vi "Upg4,5_datainsamling.vi"() -> ()   [LabVIEW 2024]
panel:
  out "Mätvärden":dbl[](array[numeric])
  in  "stanna pump":bool
  in  "Samplingsintervall (ms)":dbl
  in  "avsluta mätning":bool
  in  "Konstant (m/V)":dbl
  # "Skriv in konstant bestämd i upg 3"
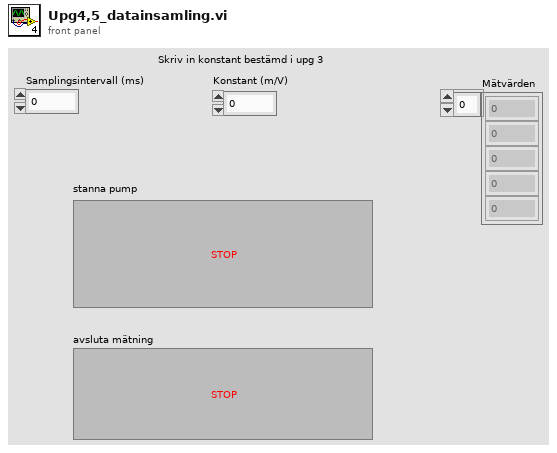
[diagram p1: front panel]
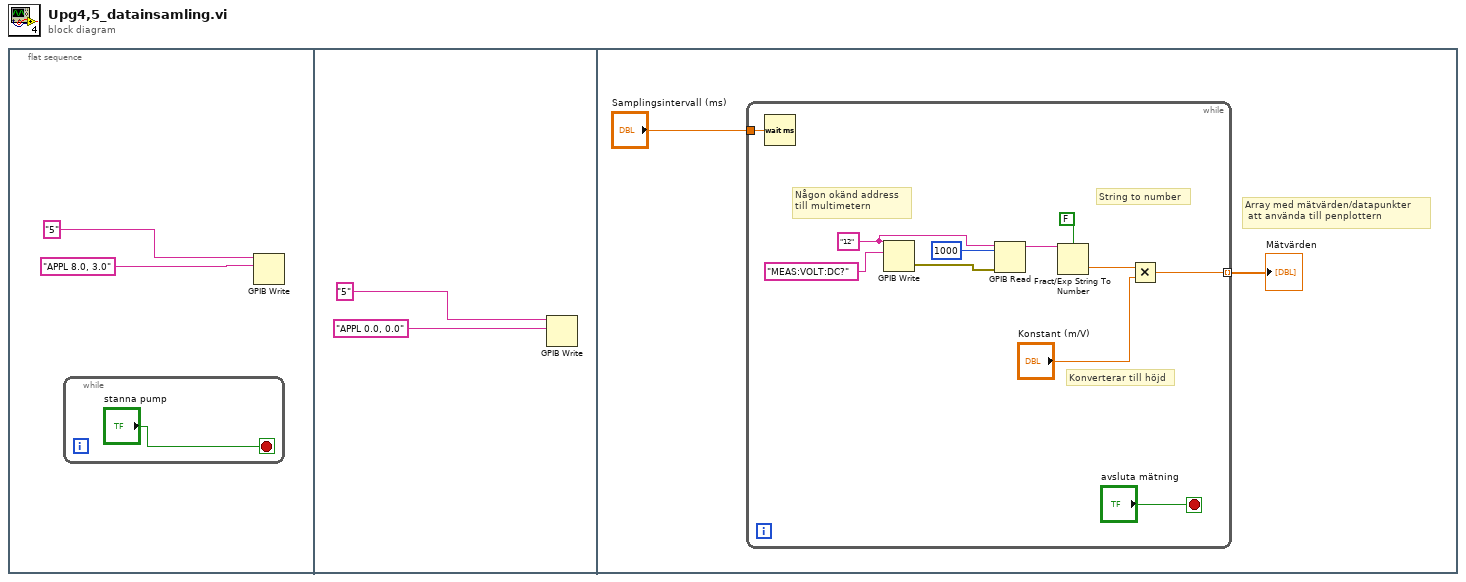
[diagram p0: block diagram]
diagram:
  n1 = flat-sequence {
    frame #0 {
      n2 = while {
        stop <- "stanna pump" stop-if-true
      }
      n3 = GPIB Write(0:"5" ("address string"), 1:"APPL 8.0, 3.0" ("data")) -> ()  [unwired: 3 in, 2 out]
    }
    frame #1 {
      n4 = GPIB Write(0:"5" ("address string"), 1:"APPL 0.0, 0.0" ("data")) -> ()  [unwired: 3 in, 2 out]
    }
    frame #2 {
      # "Array med mätvärden/datapunkter\n att använda till penplottern"
      n5 = while {
        tunnel: [w11] -> w6 mode=indexing
        tunnel: "Samplingsintervall (ms)" -> [w9]
        stop <- "avsluta mätning" stop-if-true
        w16 = "12" ("address string")
        # "Konverterar till höjd"
        # "String to number"
        # "Någon okänd address\ntill multimetern"
        n6 = Wait (ms)(milliseconds to wait=w9) -> ()  [unwired: 1 out]
        n7 = GPIB Write(0:w16, 1:"MEAS:VOLT:DC?" ("data")) -> (6:w17:errorcluster)  [unwired: 3 in, 1 out]
        n8 = GPIB Read(0:w16, 1:1000 ("byte count"), 3:w17) -> (5:w18:string)  [unwired: 2 in, 2 out]
        n9 = Fract/Exp String To Number(use system decimal point (T)=FALSE, string=w18) -> (number=w13:dbl)  [unwired: 2 in, 1 out]
        n10 = Multiply(x=w13, y="Konstant (m/V)") -> (x*y=w11:dbl)
      }
      "Mätvärden" <- w6
    }
  }
